vi "Synchonize Relay States.vi"(8 "error in (no error)":errorcluster, 11 "SLSC Switch in":refnum<class "SLSC Switch.lvclass">) -> (0 "error out":errorcluster, 3 "SLSC Switch out":refnum<class "SLSC Switch.lvclass">)   [LabVIEW 2016, in "SLSC Switch.lvlib" / "SLSC Switch.lvclass"]
uses:
  SLSC Switch.lvclass
  SLSC Switch.lvclass/SLSC Switch.ctl
  Relay/Relay.lvclass/Relay.ctl
  Switch Action Processor/Switch Action Processor.lvclass
  slscsl/slscsl.lvclass
  Relay/Relay.lvclass
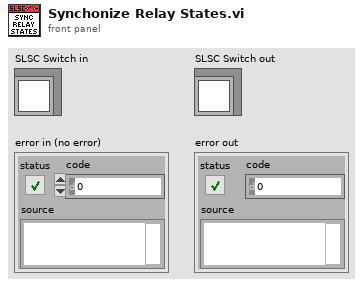
[diagram p1: front panel]
types:
  T1 = typedef "SLSC Switch.lvlib/slscsl.lvclass/RelayPosition.ctl" = i32
  T2 = typedef "SLSC Switch.lvlib/slscsl.lvclass/RelayAction.ctl" = u32
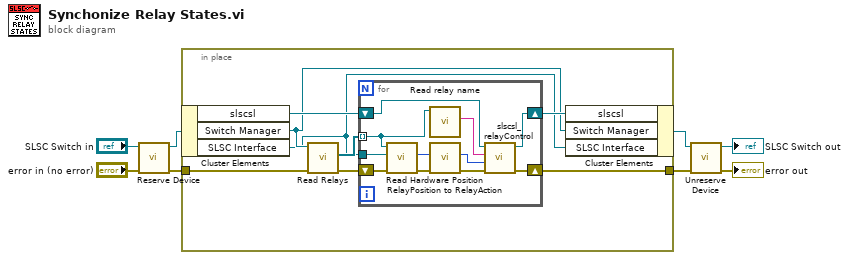
[diagram p0: block diagram]
diagram:
  n1 = call "Reserve Device.vi"("error in (no error)"="error in (no error)", "SLSC Switch in"="SLSC Switch in") -> ("error out"=w3:errorcluster, "SLSC Switch out"=w4:refnum<class "SLSC Switch.lvclass">)  [unwired: 8 in]
  n2 = in-place {
    in-place-border: [w16] -> w6
    in-place-border: w3 -> [w11]
    n3 = in-place-cluster #1(w4) -> ("slscsl"=w15:refnum<class "slscsl.lvclass">, "Switch Manager"=w12:refnum<class "Switch Action Processor.lvclass">, "SLSC Interface"=w9:refnum<class "SLSC Interface.lvclass">)
    n4 = call-dynamic "Read Relays.vi"("error in (no error)"=w11, "Switch Action Processor in"=w12) -> ("error out"=w10:errorcluster, "Relays"=w13:refnum<class "Relay.lvclass">[])  [unwired: 7 in, 1 out]
    n5 = for {
      tunnel: w13 -> [w22] mode=indexing
      shift-right: [w25] -> w14
      shift-left: w15 -> [w26]
      shift-right: [w24] -> w16
      shift-left: w10 -> [w20]
      tunnel: w9 -> [w17]
      n6 = call "Read Hardware Position.vi"("error in (no error)"=w20, "SLSC Session In"=w17, "Relay in"=w22) -> ("error out"=w18:errorcluster, "RelayPosition"=w19:T1)  [unwired: 6 in, 1 out]
      n7 = call "Read relay name.vi"("Relay in"=w22) -> ("name"=w21:string)  [unwired: 8 in, 2 out]
      n8 = call "RelayPosition to RelayAction.vi"("position"=w19) -> ("action"=w23:T2)  [unwired: 10 in]
      n9 = call "slscsl_relayControl.vi"("error in (no error)"=w18, "RelayAction"=w23, "relayNames"=w21, "slscsl in"=w26) -> ("error out"=w24:errorcluster, "slscsl out"=w25:refnum<class "slscsl.lvclass">)  [unwired: 5 in, 1 out]
    }
    n10 = in-place-cluster #1("slscsl"=w14, "Switch Manager"=w12, "SLSC Interface"=w9) -> (w5:refnum<class "SLSC Switch.lvclass">)
  }
  n11 = call "Unreserve Device.vi"("error in (no error)"=w6, "SLSC Switch in"=w5) -> ("error out"=→"error out":errorcluster, "SLSC Switch out"=→"SLSC Switch out":refnum<class "SLSC Switch.lvclass">)  [unwired: 8 in]
